vi "YKMW100 RW Math Constants.vi"(0 "MW100":refnum<visa-resource-name>="MW100", 2 "Semiphore":T1, 5 "Channel_Enum":T2=38 items=["4-20_OUT", "Pres_HI1", "Pres_HI2", "Pres_LOW", "Pres_PIN", "HEATER_TOP", "HEATER_BOT", "T_Shell", "FLOWMETER", "WATT_SENSE", "WH_TICK", "Tc_1", "Tc_2", "Tc_3", "Tc_4", "Tc_5", "Tc_6", "Tc_down", "T_Shell_2", "T_Shell_3", "T_Shell_4", "RTD_IN", "RTD_OUT", "RTD_AMB", "INTF_TEMPFLO", "INTF_READY", "INTF_START", "INTF_STOP", "DRM_LOW", "DRM_HIGH", "PWR_MAIN", "VLV_DUMP", "VLV_OUT", "VLV_IN", "WATT_HOURS", "FLOW(SAMPLE)", "GALLONS", "FLOW(GPM)", "FLOW_CALC_GAIN", "FLOW_CALC_OFFSET", "FLOW_CALC_THRESHOLD"], 7 "Write Value":string, 9 "Read? (Write=F)":bool, 11 "Error In":errorcluster) -> (4 "dup VISA session":refnum<visa-resource-name>, 6 "Read Value":dbl, 15 "Error Out":errorcluster)   [LabVIEW 2009]
uses:
  ChannelSettings.ctl
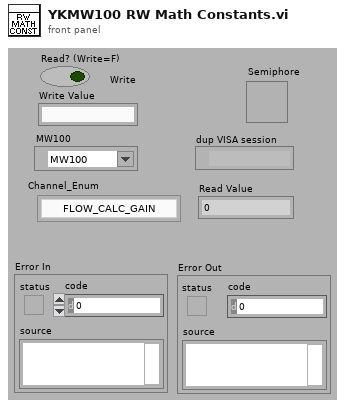
[diagram p1: front panel]
types:
  T1 = typedef "Semaphore RefNum" = refnum<k1>
  T2 = typedef "ChannelSettings.ctl" = u32
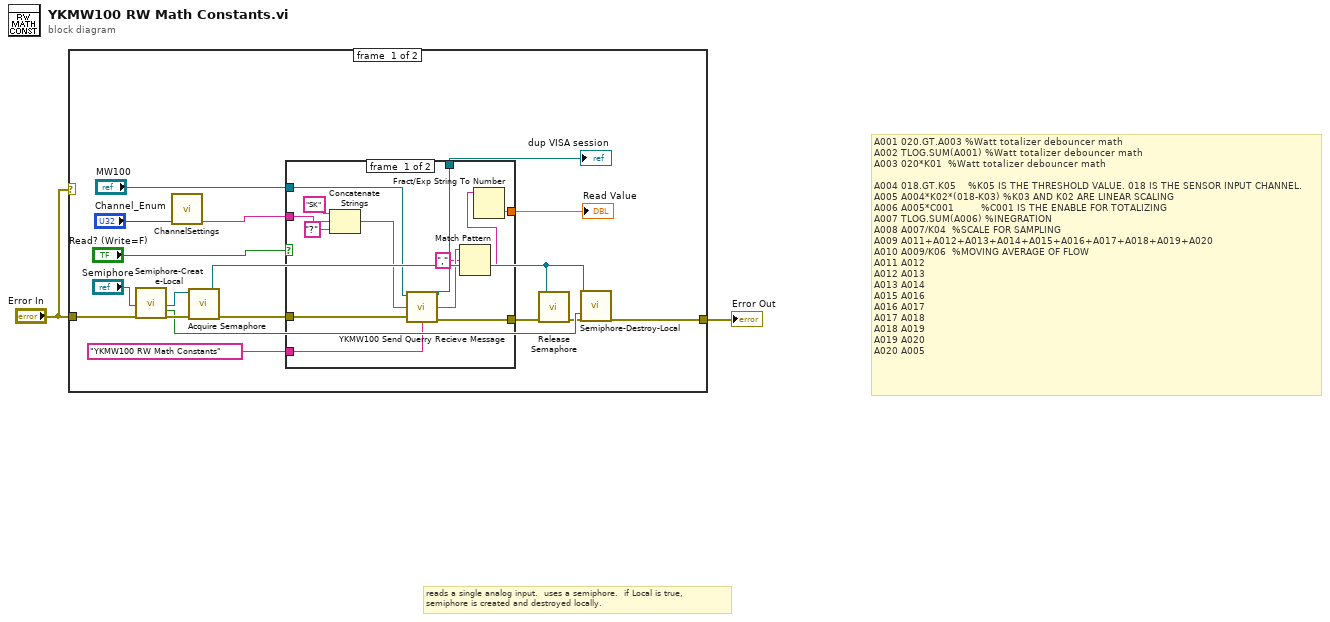
[diagram p0: block diagram]
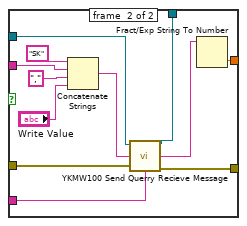
[diagram p2: hidden frame]
diagram:
  # "A001 020.GT.A003\t%Watt totalizer debouncer math\nA002 TLOG.SUM(A001)\t%Watt totalizer debouncer math\nA003 020*K01\t\t%Watt totalizer debouncer math\n\nA004 018.GT.K05   \t%K05 IS THE THRESHOLD VALUE. 018 IS THE SENSOR INPUT CHANNEL.\nA005 A004*K02*(018-K03) %K03 AND K02 ARE LINEAR SCALING\nA006 A005*C001        \t%C001 IS THE ENABLE FOR TOTALIZING\nA007 TLOG.SUM(A006)\t%INEGRATION\nA008 A007/K04\t\t%SCALE FOR SAMPLING\nA009 A011+A012+A013+A014+A015+A016+A017+A018+A019+A020\nA010 A009/K06\t\t%MOVING AVERAGE OF FLOW\nA011 A012\nA012 A013\nA013 A014\nA015 A016\nA016 A017\nA017 A018\nA018 A019\nA019 A020\nA020 A005"
  # "reads a single analog input.  uses a semiphore.  if Local is true, \nsemiphore is created and destroyed locally."
  n1 = case shown="No Error" "Error In" {
    tunnel: "Error In" -> [w17 w45]
    tunnel: [w11 w45] -> w2
    frame #0 {
      n2 = call "Semiphore-Create-Local.vi"("Semiphore"="Semiphore", "error in (no error)"=w17) -> ("semaphore"=w16:T1, "Local?"=w13:bool, "error out"=w15:errorcluster)  [unwired: 15 in]
      n3 = call "ChannelSettings.vi"("Channel_Enum"="Channel_Enum") -> ("Channel String"=w5:string)  [unwired: 10 in]
      n4 = call <vilib>:"Acquire Semaphore.vi"("error in (no error)"=w15, "semaphore"=w16) -> ("error out"=w7:errorcluster, "semaphore out"=w14:T1)  [unwired: 3 in, 1 out]
      n5 = case shown="True" "Read? (Write=F)" {
        tunnel: "MW100" -> [w32 w44]
        tunnel: [w31 w43] -> w9
        tunnel: "YKMW100 RW Math Constants" ("Source (\"\")") -> [w30 w42]
        tunnel: w7 -> [w29 w41]
        tunnel: [w28 w40] -> w6
        tunnel: w5 -> [w26 w38]
        tunnel: [w23 w34] -> w4
        frame #0 {
          n6 = Concatenate Strings("SK" ("string"), w26, "?" ("string")) -> (w24:string)
          n7 = call "YKMW100 Send Querry Recieve Message.vi"("VISA session"=w32, "Send Message (\"\")"=w24, "error in (no error)"=w29, "Source (\"\")"=w30) -> ("dup VISA session"=w31:refnum<visa-resource-name>, "Read Buffer"=w22:string, "error out"=w28:errorcluster)  [unwired: 9 in]
          n8 = Match Pattern(string=w22, regular expression=",") -> (after substring=w20:string)  [unwired: 1 in, 3 out]
          n9 = Fract/Exp String To Number(string=w20) -> (number=w23:dbl)  [unwired: 3 in, 1 out]
        }
        frame #1 {
          n10 = Concatenate Strings("SK" ("string"), w38, "," ("string"), "Write Value") -> (w36:string)
          n11 = call "YKMW100 Send Querry Recieve Message.vi"("VISA session"=w44, "Send Message (\"\")"=w36, "error in (no error)"=w41, "Source (\"\")"=w42) -> ("dup VISA session"=w43:refnum<visa-resource-name>, "Read Buffer"=w35:string, "error out"=w40:errorcluster)  [unwired: 9 in]
          n12 = Fract/Exp String To Number(string=w35) -> (number=w34:dbl)  [unwired: 3 in, 1 out]
        }
      }
      "Read Value" <- w4
      "dup VISA session" <- w9
      n13 = call <vilib>:"Release Semaphore.vi"("error in (no error)"=w6, "semaphore"=w14) -> ("error out"=w12:errorcluster)  [unwired: 4 in, 1 out]
      n14 = call "Semiphore-Destroy-Local.vi"("Semiphore"=w14, "Local?"=w13, "error in (no error)"=w12) -> ("error out"=w11:errorcluster)  [unwired: 16 in]
    }
    frame #1 {
    }
  }
  "Error Out" <- w2
